vi "stepper_getpos.vi"(8 "error in (no error)":errorcluster, 11 "reference":refnum<k7>) -> (0 "error out":errorcluster, 2 "pfPosition[µm]":sgl, 3 "reference out":refnum<k7>)   [LabVIEW 2018]
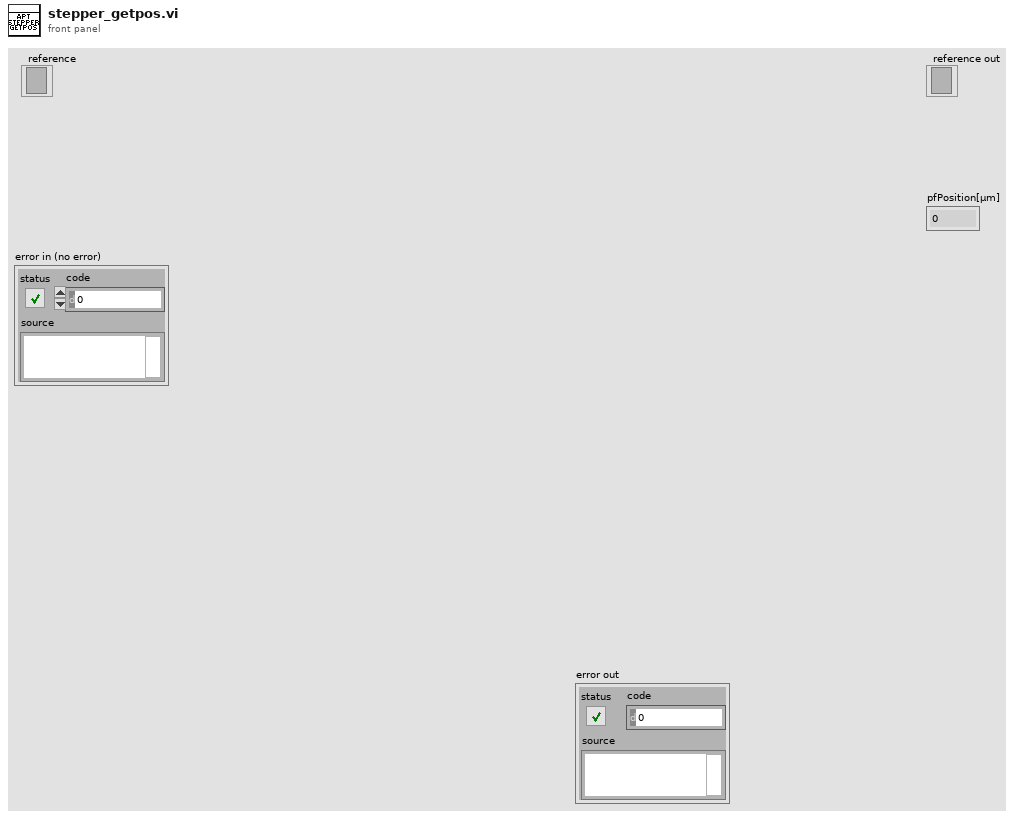
[diagram p1: front panel]
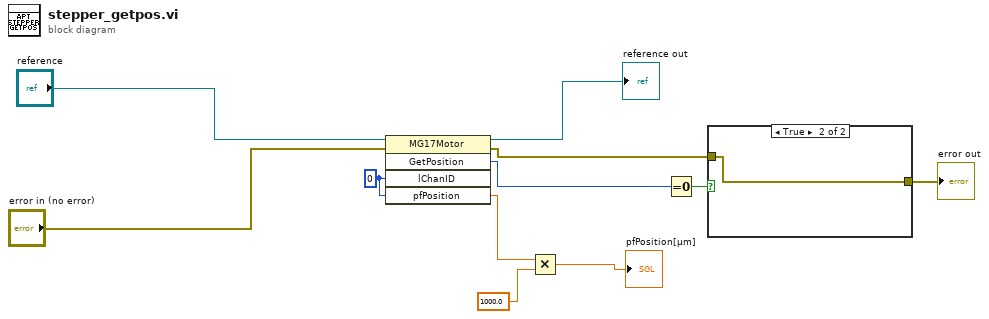
[diagram p0: block diagram]
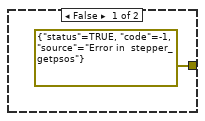
[diagram p2: hidden frame]
diagram:
  w9 = 0 ("lChanID")
  n1 = invoke class="MG17Motor" method="GetPosition"(reference="reference", error in="error in (no error)", "lChanID"=w9, "pfPosition"=w9) -> (reference out=→"reference out":refnum<k7>, error out=w1:errorcluster, "GetPosition"=w2:i32, "pfPosition"=w7:sgl)  [unwired: 1 in, 1 out]
  n2 = Multiply(x=w7, y=sgl 1000.0) -> (x*y=→"pfPosition[µm]":sgl)
  n3 = Equal To 0?(x=w2) -> (x = 0?=w4:bool)
  n4 = case shown="True" w4 {
    tunnel: [errorcluster {"status"=TRUE, "code"=-1, "source"="Error in  stepper_getpsos"} ("error out") w13] -> w3
    tunnel: w1 -> [_ w13]
    frame False {
    }
    frame True {
    }
  }
  "error out" <- w3
